vi "Write Stiffnesses Data Summary.vi"(10 "Stiffnesses Data Summary":T1 {"Forces" min=-888.0 max=888.0; "Stiffnesses" min=-199630324.20594117 max=199630324.20594117 format="%.2f"; "Displacements" min=-0.19963032420594115 max=0.19963032420594115 format="%.2f"}, 11 "TestDataLog in":refnum<class "TestDataLog.lvclass">) -> (3 "TestDataLog out":refnum<class "TestDataLog.lvclass">)   [LabVIEW 2015, in "TestDataLog.lvclass"]
uses:
  TestDataLog.lvclass
  Typedefs/StiffnessesDataSummary.ctl
  TestDataLog.lvclass/TestDataLog.ctl
  Typedefs/M1M3SSSTypedefs.lvlib
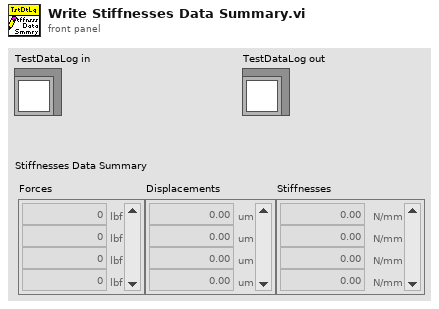
[diagram p1: front panel]
types:
  T1 = typedef "M1M3SSSTypedefs.lvlib/StiffnessesDataSummary.ctl" = cluster{"Forces":dbl[unit][], "Displacements":dbl[unit][], "Stiffnesses":dbl[unit][]}
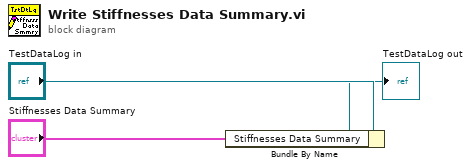
[diagram p0: block diagram]
diagram:
  n1 = Bundle By Name(cluster="TestDataLog in", "Stiffnesses Data Summary"="Stiffnesses Data Summary") -> (→"TestDataLog out":refnum<class "TestDataLog.lvclass">)
